vi "Update Dynamic Configurations.vi"(6 "Write Ref":T2, 7 "Read Write Ref":T1, 8 "error in":errorcluster, 10 "AsyncRequest":T4, 11 "Compiled.Settings in":T3) -> (0 "error out":errorcluster, 2 "Response Ref":refnum<queue>, 3 "Compiled.Settings out":T3)   [LabVIEW 2026, in "Runtime Configuration Support Inline Async Example Custom Device Engine.lvlib"]
uses:
  Runtime Configuration Support Inline Async Example Custom Device Engine.lvlib
  Shared/Compiled.Settings.ctl
  AsyncRequest.ctl
  <vilib>/NI/NIVS Inline Async API/_Data Access Engine/Data Access Engine/Types/Write.DVR.ctl
  <vilib>/NI/NIVS Inline Async API/_Data Access Engine/Access Type Classes/Write/Write.lvclass
  <vilib>/NI/NIVS Inline Async API/_Data Access Engine/Data Access Engine/Types/ReadWrite.DVR.ctl
  <vilib>/NI/NIVS Inline Async API/_Data Access Engine/Access Type Classes/ReadWrite/ReadWrite.lvclass
  Shared/Runtime Configuration Support Inline Async Example Custom Device Shared.lvlib
  <vilib>/NI/NIVS Inline Async API/_Data Access Engine/Data Access Engine/Data Access Engine.lvclass
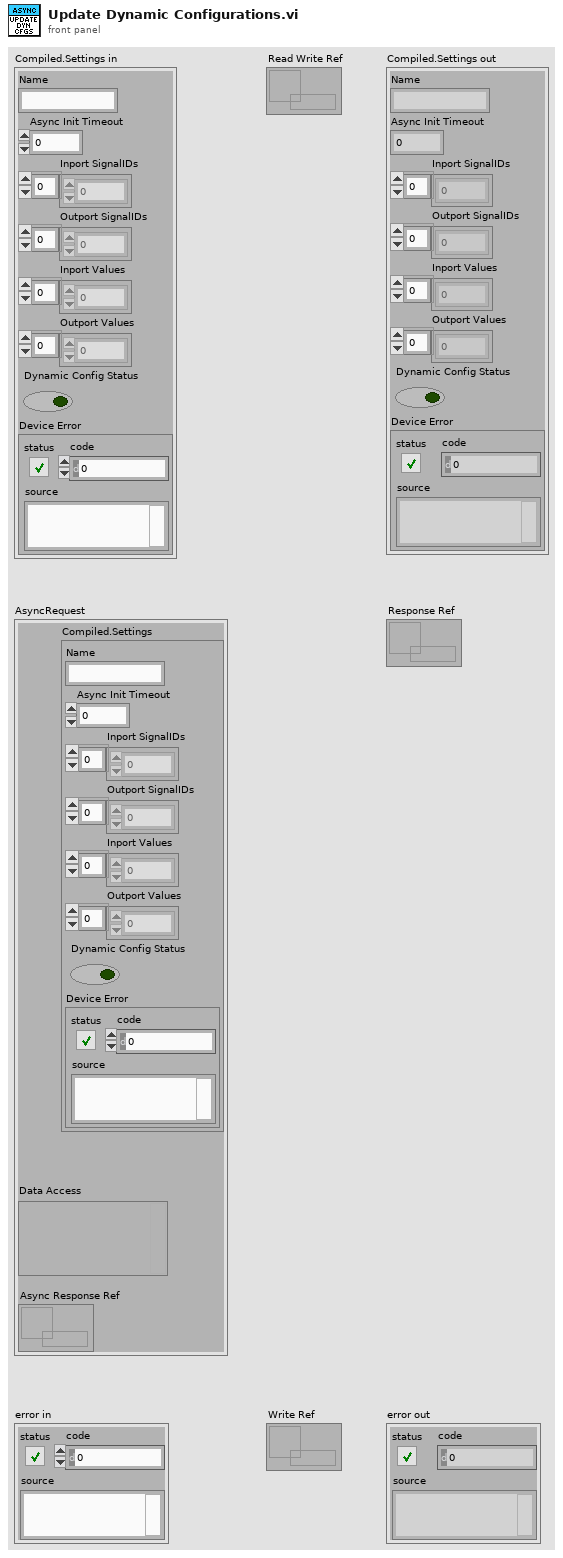
[diagram p1: front panel]
types:
  T1 = typedef "Data Access Engine.lvlib/Data Access Engine.lvclass/ReadWrite.DVR.ctl" = refnum<data-value>
  T2 = typedef "Data Access Engine.lvlib/Data Access Engine.lvclass/Write.DVR.ctl" = refnum<data-value>
  T3 = typedef "Runtime Configuration Support Inline Async Example Custom Device Shared.lvlib/Compiled.Settings.ctl" = cluster{"Name":string, "Async Init Timeout":u16, "Inport SignalIDs":i32[], "Outport SignalIDs":i32[], "Inport Values":dbl[], "Outport Values":dbl[], "Dynamic Config Status":bool, "Device Error":errorcluster}
  T4 = typedef "Runtime Configuration Support Inline Async Example Custom Device Engine.lvlib/AsyncRequest.ctl" = cluster{"Compiled.Settings":T3, "Data Access":variant, "Async Response Ref":refnum<queue>}
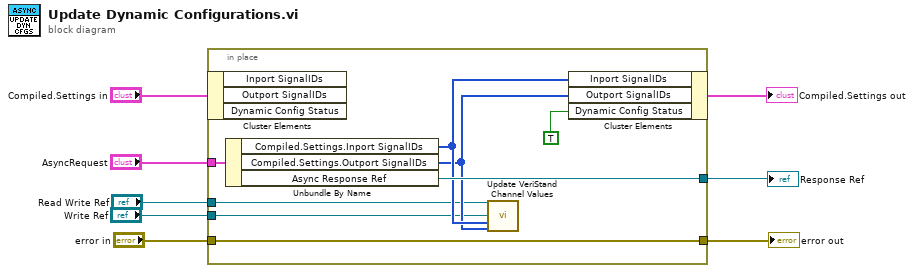
[diagram p0: block diagram]
diagram:
  n1 = in-place {
    in-place-border: "AsyncRequest" -> [w15]
    in-place-border: [w14] -> w4
    in-place-border: "error in" -> [w16]
    in-place-border: [w16] -> w7
    in-place-border: "Write Ref" -> [w10]
    in-place-border: "Read Write Ref" -> [w9]
    n2 = in-place-cluster #1("Compiled.Settings in") -> ()  [unwired: 3 out]
    n3 = Unbundle By Name(w15) -> ("Compiled.Settings.Inport SignalIDs"=w12:i32[], "Compiled.Settings.Outport SignalIDs"=w11:i32[], "Async Response Ref"=w14:refnum<queue>)
    n4 = call "Update VeriStand Channel Values.vi"("SignalIds Out"=w11, "SignalIds In"=w12, "Write Ref"=w10, "Read Write Ref"=w9) -> ()  [unwired: 8 in]
    n5 = in-place-cluster #1("Inport SignalIDs"=w12, "Outport SignalIDs"=w11, "Dynamic Config Status"=TRUE) -> (→"Compiled.Settings out":T3)
  }
  "Response Ref" <- w4
  "error out" <- w7
